vi "Working Graph Model.vi"() -> ()   [LabVIEW 2015]
uses:
  <vilib>/addons/Control Design/_Model Construction/Data Typedefs.llb/CD Time Info.ctl
  <vilib>/addons/JSON API/JSON Value/Set from JSON string.vi
  <vilib>/addons/JSON API/JSON Value/Get Object Item by Name.vi
  <vilib>/addons/JSON API/JSON Scalar/Get as DBL.vi
  <vilib>/addons/Control Design/_Model Construction/Model Creation.llb/Model Creation SubVI/cd_Create Symbolic Transfer Function Model.vi
  <vilib>/addons/Control Design/_Utility/Model Viewer.llb/Model Viewer SubVI/cd_Draw Transfer Function Equation (TF).vi
  <vilib>/addons/Control Design/_Time Response Analysis/Time Response.llb/Time Response subVI/cd_Step Response (Transfer Function).vi
  <vilib>/addons/JSON API/JSON Value/JSON Value.lvclass
  <vilib>/addons/Control Design/_Model Construction/NI_LinSys_Model Creation.lvlib
  <vilib>/addons/Control Design/_Utility/NI_CD_Model Viewer.lvlib
  <vilib>/addons/Control Design/_Time Response Analysis/NI_CD_Time Response.lvlib
  <vilib>/addons/JSON API/Get Polymorphic/JSON GetSet.lvlib
  <vilib>/addons/JSON API/JSON Scalar/JSON Scalar.lvclass
  <vilib>/addons/Control Design/_Model Construction/NI_LinSys_Data Typedefs.lvlib
panel:
  out "output array":dbl[](array[numeric])
  out "Final Output Data":string
  out "Time":string
  out "Data String":string
  out "Step Response Graph 2":cluster{"time":dbl[], dbl[]}[](graph)
  out "Equation 2":picture
  out "Processed":string
  out "error out":errorcluster
  out "F":dbl
  out "Vin 2":dbl
  out "D":dbl
  out "L":dbl
  out "C":dbl
  out "R":dbl
  out "r1":dbl
  in  "stop":bool
  out "In":string
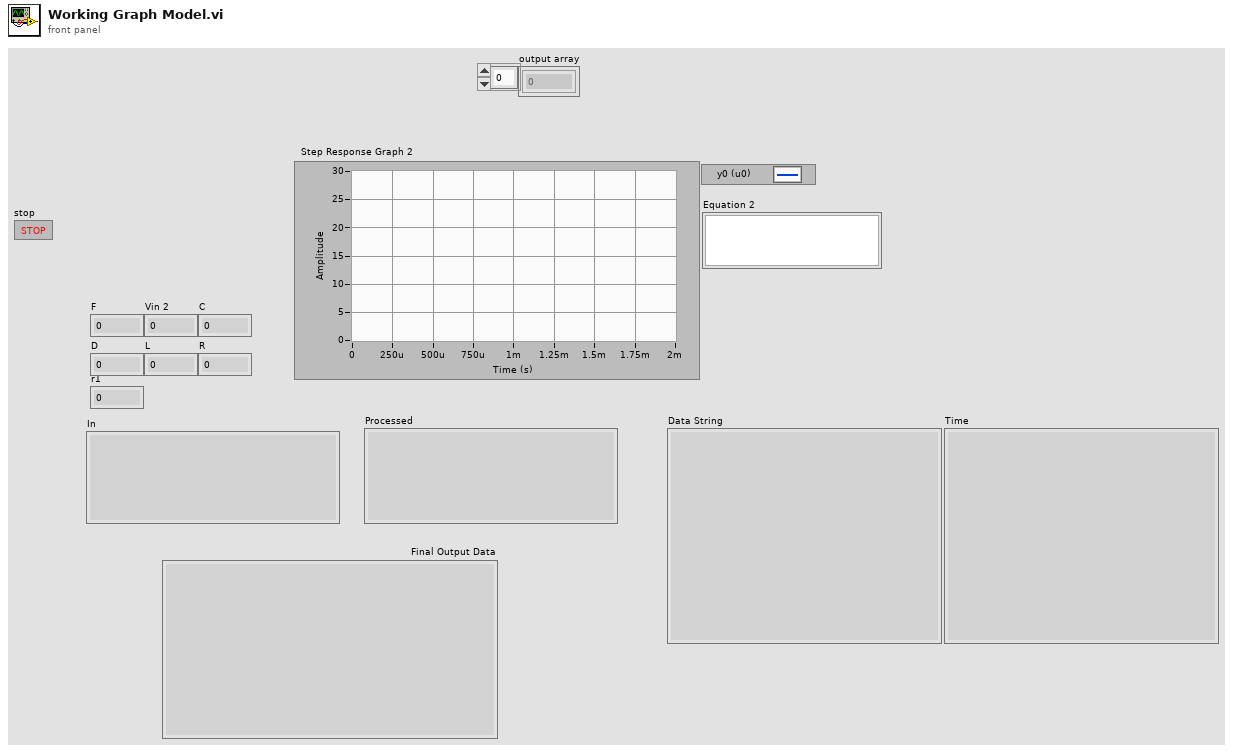
[diagram p1: front panel]
types:
  T1 = typedef "NI_LinSys_Data Typedefs.lvlib/CD Time Info.ctl" = cluster{"t0":dbl, "dt":dbl, "tf":dbl}
  T2 = typedef "NI_LinSys_Model Typedefs.lvlib/CD Transfer Function Model (MIMO).ctl" = cluster{"properties":T3, "transfer function(s)":T4[][]}
  T3 = typedef "NI_LinSys_Model Typedefs.lvlib/CD General Elements.ctl" = cluster{"Model name":string, "Input names":string[], "Output names":string[], "Input Delays":dbl[], "Output Delays":dbl[], "Sampling Time":dbl, "Notes":string}
  T4 = typedef "NI_LinSys_Model Typedefs.lvlib/CD Transfer Function Model (SISO).ctl" = cluster{"Numerator":dbl[], "Denominator":dbl[], "delay":dbl}
  T5 = typedef "NI_LinSys_Data Typedefs.lvlib/CD MIMO Time Response Data.ctl" = cluster{"Time":dbl[], "Outputs Data":dbl[][][], "States Data":dbl[][][], "plot type":T6}
  T6 = typedef "NI_LinSys_Data Typedefs.lvlib/CD Plot Types Enum.ctl" = enum16{"bode-magnitude", "bode-phase", "nichols", "nyquist", "singular values", "step", "impulse", "initial", "simulation", "nyquist with separation"}
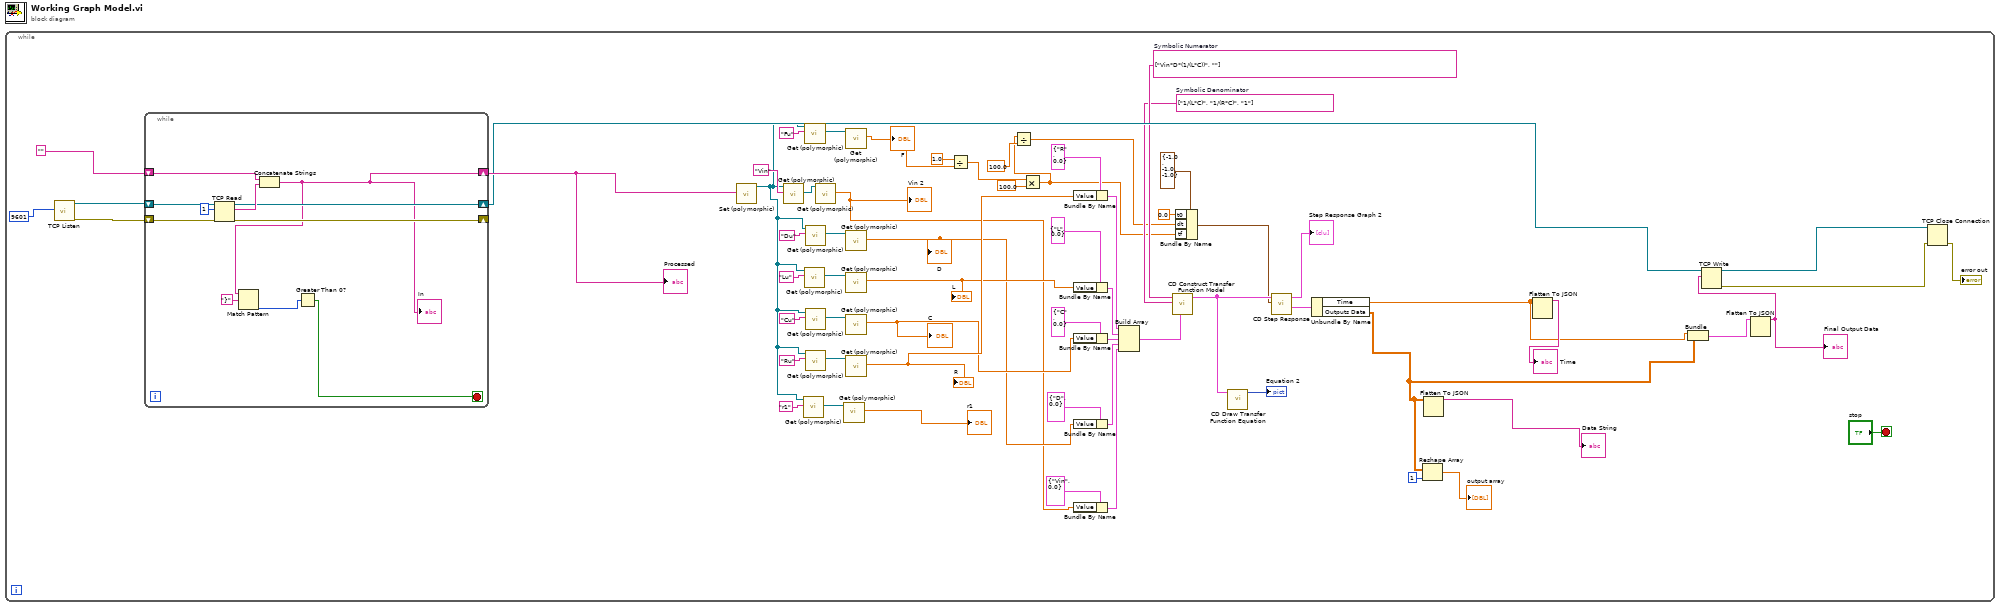
[diagram p0: block diagram]
diagram:
  n1 = while {
    stop <- "stop" stop-if-true
    w39 = string[] ["1/(L*C)", "1/(R*C)", "1"]  # Symbolic Denominator
    w40 = string[] ["Vin*D*(1/(L*C))", ""]  # Symbolic Numerator
    n2 = call <vilib>:"TCP Listen.vi"("port"=u16 9601) -> ("error out"=w64:errorcluster, "connection ID"=w63:refnum<k5>)  [unwired: 6 in, 3 out]
    n3 = while {
      shift-right: [w70] -> w50
      shift-left: "" -> [w77]
      shift-right: [w74] -> _
      shift-left: w64 -> [w76]
      shift-right: [w71] -> w46
      shift-left: w63 -> [w75]
      stop <- w67 stop-if-true
      n4 = TCP Read(connection ID=w75, bytes to read=1, error in (no error)=w76) -> (connection ID out=w71:refnum<k5>, data out=w72:string, error out=w74:errorcluster)  [unwired: 2 in]
      n5 = Concatenate Strings(w77, w72) -> (w70:string)
      "In" <- w70
      n6 = Match Pattern(string=w70, regular expression="}") -> (offset past match=w68:i32)  [unwired: 1 in, 3 out]
      n7 = Greater Than 0?(x=w68) -> (x > 0?=w67:bool)
    }
    "Processed" <- w50
    n8 = call-poly <vilib>:"Set (polymorphic).vi"("JSON stream"=w50) -> ("JSON Value out"=w43:refnum<class "JSON Value.lvclass">)  [unwired: 8 in, 2 out]
    n9 = call-poly <vilib>:"Get (polymorphic).vi"("name"="Vin", "JSON Value In"=w43) -> ("Value"=w61:refnum<class "JSON Value.lvclass">)  [unwired: 6 in, 3 out]
    n10 = call-poly <vilib>:"Get (polymorphic).vi"("name"="r1", "JSON Value In"=w43) -> ("Value"=w45:refnum<class "JSON Value.lvclass">)  [unwired: 6 in, 3 out]
    n11 = call-poly <vilib>:"Get (polymorphic).vi"("name"="Lu", "JSON Value In"=w43) -> ("Value"=w58:refnum<class "JSON Value.lvclass">)  [unwired: 6 in, 3 out]
    n12 = call-poly <vilib>:"Get (polymorphic).vi"("name"="Fu", "JSON Value In"=w43) -> ("Value"=w52:refnum<class "JSON Value.lvclass">)  [unwired: 6 in, 3 out]
    n13 = call-poly <vilib>:"Get (polymorphic).vi"("name"="Du", "JSON Value In"=w43) -> ("Value"=w60:refnum<class "JSON Value.lvclass">)  [unwired: 6 in, 3 out]
    n14 = call-poly <vilib>:"Get (polymorphic).vi"("name"="Cu", "JSON Value In"=w43) -> ("Value"=w56:refnum<class "JSON Value.lvclass">)  [unwired: 6 in, 3 out]
    n15 = call-poly <vilib>:"Get (polymorphic).vi"("name"="Ru", "JSON Value In"=w43) -> ("Value"=w54:refnum<class "JSON Value.lvclass">)  [unwired: 6 in, 3 out]
    n16 = call-poly <vilib>:"Get (polymorphic).vi"("JSON Value in"=w61) -> ("Number"=w14:dbl)  [unwired: 8 in, 2 out]
    "Vin 2" <- w14
    n17 = call-poly <vilib>:"Get (polymorphic).vi"("JSON Value in"=w45) -> ("Number"=→"r1":dbl)  [unwired: 8 in, 2 out]
    n18 = call-poly <vilib>:"Get (polymorphic).vi"("JSON Value in"=w52) -> ("Number"=w12:dbl)  [unwired: 8 in, 2 out]
    "F" <- w12
    n19 = call-poly <vilib>:"Get (polymorphic).vi"("JSON Value in"=w60) -> ("Number"=w15:dbl)  [unwired: 8 in, 2 out]
    "D" <- w15
    n20 = call-poly <vilib>:"Get (polymorphic).vi"("JSON Value in"=w58) -> ("Number"=w17:dbl)  [unwired: 8 in, 2 out]
    "L" <- w17
    n21 = call-poly <vilib>:"Get (polymorphic).vi"("JSON Value in"=w56) -> ("Number"=w16:dbl)  [unwired: 8 in, 2 out]
    "C" <- w16
    n22 = call-poly <vilib>:"Get (polymorphic).vi"("JSON Value in"=w54) -> ("Number"=w18:dbl)  [unwired: 8 in, 2 out]
    "R" <- w18
    n23 = Divide(x=1.0, y=w12) -> (x/y=w6:dbl)
    n24 = Multiply(x=w6, y=100.0) -> (x*y=w5:dbl)
    n25 = Divide(x=w5, y=100.0) -> (x/y=w8:dbl)
    n26 = Bundle By Name(cluster=cluster{"Name":string, " Value":dbl} {"Name"="R", " Value"=0.0} ("input cluster"), "Value"=w18) -> (w33:cluster{"Name":string, " Value":dbl})
    n27 = Bundle By Name(cluster=cluster{"Name":string, " Value":dbl} {"Name"="L", " Value"=0.0} ("Variable 2"), "Value"=w17) -> (w32:cluster{"Name":string, " Value":dbl})
    n28 = Bundle By Name(cluster=cluster{"Name":string, " Value":dbl} {"Name"="C", " Value"=0.0} ("Variable"), "Value"=w16) -> (w31:cluster{"Name":string, " Value":dbl})
    n29 = Bundle By Name(cluster=cluster{"Name":string, " Value":dbl} {"Name"="D", " Value"=0.0} ("Variable"), "Value"=w15) -> (w30:cluster{"Name":string, " Value":dbl})
    n30 = Bundle By Name(cluster=cluster{"Name":string, " Value":dbl} {"Name"="Vin", " Value"=0.0} ("Variable"), "Value"=w14) -> (w24:cluster{"Name":string, " Value":dbl})
    n31 = Build Array(w33, w32, w31, w30, w24) -> (w29:cluster{"Name":string, " Value":dbl}[])
    n32 = call-poly <vilib>:"CD Construct Transfer Function Model.vi"("Variables"=w29, "Symbolic Denominator"=w39, "Symbolic Numerator"=w40) -> ("Transfer Function Model"=w27:T2)  [unwired: 7 in, 1 out]
    n33 = Bundle By Name(cluster=T1 {"t0"=-1.0, "dt"=-1.0, "tf"=-1.0} ("Time Range"), "t0"=0.0, "dt"=w8, "tf"=w5) -> (w7:T1)
    n34 = call-poly <vilib>:"CD Draw Transfer Function Equation.vi"("Transfer Function Model"=w27) -> ("Equation"=→"Equation 2":picture)  [unwired: 8 in, 2 out]
    n35 = call-poly <vilib>:"CD Step Response.vi"("Time Range"=w7, "Transfer Function Model"=w27) -> ("Step Response Data"=w26:T5, "Step Response Graph"=→"Step Response Graph 2":cluster{"time":dbl[], dbl[]}[])  [unwired: 7 in, 1 out]
    n36 = Unbundle By Name(w26) -> ("Time"=w21:dbl[], "Outputs Data"=w3:dbl[][][])
    n37 = Reshape Array(w3, 1 ("dimension size")) -> (→"output array":dbl[])
    n38 = Flatten To JSON(anything=w3) -> (JSON string=→"Data String":string)  [unwired: 2 in, 1 out]
    n39 = Flatten To JSON(anything=w21) -> (JSON string=→"Time":string)  [unwired: 2 in, 1 out]
    n40 = Bundle("Time"=w21, "Outputs Data"=w3) -> (w20:cluster{"Time":dbl[], "Outputs Data":dbl[][][]})  [unwired: 1 in]
    n41 = Flatten To JSON(anything=w20) -> (JSON string=w19:string)  [unwired: 2 in, 1 out]
    "Final Output Data" <- w19
    n42 = TCP Write(connection ID=w46, data in=w19) -> (connection ID out=w49:refnum<k5>, error out=w48:errorcluster)  [unwired: 2 in, 1 out]
    n43 = TCP Close Connection(connection ID=w49, error in (no error)=w48) -> (error out=→"error out":errorcluster)  [unwired: 1 in, 1 out]
  }
